vi "Static panel wrapper.vi"(6 "Fiber Auto Collimation state data":refnum<class "Fiber Auto Collimation state data.lvclass">, 7 "Station config":refnum<class "Station config.lvclass">, 8 "error in (no error)":errorcluster, 9 "Start hidden?":bool, 10 "Clone name [blank = only one instance]":string, 11 "Fiber Auto Collimation panel in":refnum<class "Fiber Auto Collimation panel.lvclass">) -> (0 "error out":errorcluster, 3 "Fiber Auto Collimation panel out":refnum<class "Fiber Auto Collimation panel.lvclass">)   [LabVIEW 2018, in "Fiber Auto Collimation panel.lvclass"]
doc: "This VI doesn't do much on its own. \n\nIt is mostly just a wrapper for the Dynamic Dispatch VI that it calls, because a \"Call by reference\" node can't call a Dynamic Dispatch VI directly.\n\nThe one things it does do besides being a wrapper is it writes the \"start hidden\" Boolean and the clone name to the Panel reference before passing it on."
uses:
  Fiber Auto Collimation panel.lvclass
  State data/Fiber Auto Collimation state data.lvclass
  <userlib>/Recipe/Station Config/Station config.lvclass
  Fiber Auto Collimation panel.lvclass/Fiber Auto Collimation panel.ctl
  <vilib>/Utility/error.llb/Trim Whitespace.vi
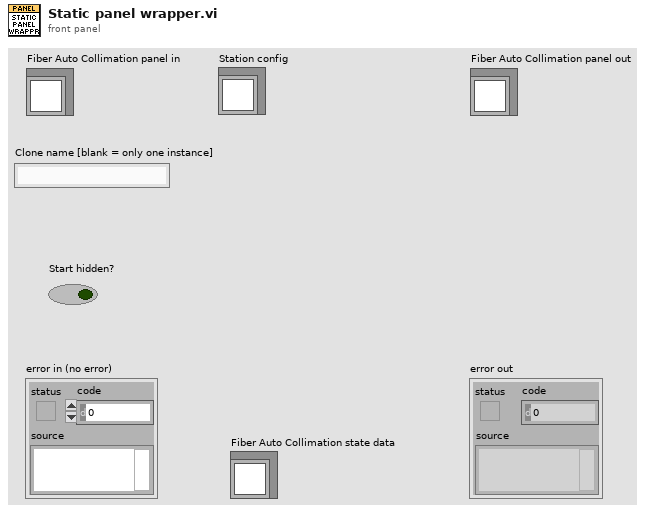
[diagram p1: front panel]
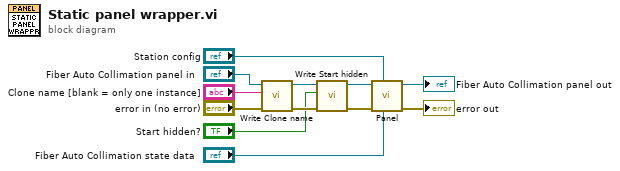
[diagram p0: block diagram]
diagram:
  n1 = call "Write Clone name.vi"("error in (no error)"="error in (no error)", "Clone name"="Clone name [blank = only one instance]", "Fiber Auto Collimation panel in"="Fiber Auto Collimation panel in") -> ("error out"=w7:errorcluster, "Fiber Auto Collimation panel out"=w3:refnum<class "Fiber Auto Collimation panel.lvclass">)  [unwired: 7 in]
  n2 = call "Write Start hidden.vi"("error in (no error)"=w7, "Start hidden"="Start hidden?", "Fiber Auto Collimation panel in"=w3) -> ("error out"=w4:errorcluster, "Fiber Auto Collimation panel out"=w2:refnum<class "Fiber Auto Collimation panel.lvclass">)  [unwired: 7 in]
  n3 = call-dynamic "Panel.vi"("Fiber Auto Collimation state data"="Fiber Auto Collimation state data", "Station config"="Station config", "error in (no error)"=w4, "Fiber Auto Collimation panel in"=w2) -> ("error out"=→"error out":errorcluster, "Fiber Auto Collimation panel out"=→"Fiber Auto Collimation panel out":refnum<class "Fiber Auto Collimation panel.lvclass">)  [unwired: 6 in]
